vi "add channel test.vi"() -> (0 "no error":errorcluster, 1 "names":string[](array[string]), 2 "channels":refnum<class "TBM channel.lvclass">[](array[class]), 3 "sample module configuration out":refnum<class "sample module configuration.lvclass">)   [LabVIEW 2013, in "sample module tests.lvlib"]
uses:
  sample module tests.lvlib
  channel/TBM channel.lvclass
  module/configuration/sample module configuration.lvclass
  channel/channel classification.ctl
  root configuration/TBM configuration.lvclass
panel:
  out "channels match":bool
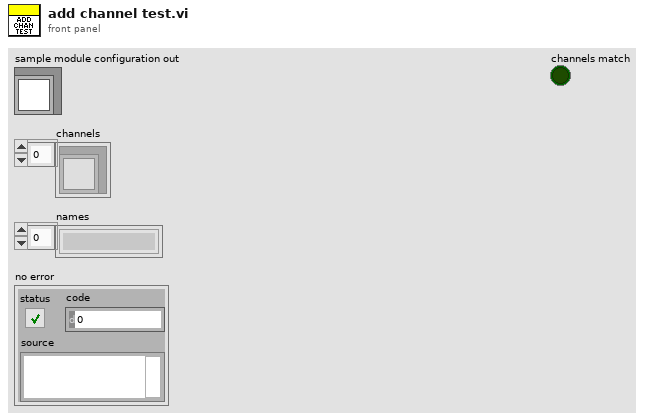
[diagram p1: front panel]
types:
  T1 = typedef "TBM channel.lvclass/channel classification.ctl" = enum16{"input data", "output data", "processing parameter", "processing result"}
  T2 = typedef "tag bus.lvlib/tag descriptor.lvclass/Data Type.ctl" = enum16{"Double", "Single", "I64", "I32", "I16", "I8", "U64", "U32", "U16", "U8", "Boolean", "String", "Array of Double", "Array of Single", "Array of I64", "Array of I32", "Array of I16", "Array of I8", "Array of U64", "Array of U32", "Array of U16", "Array of U8", "Array of Boolean", "Array of String"}
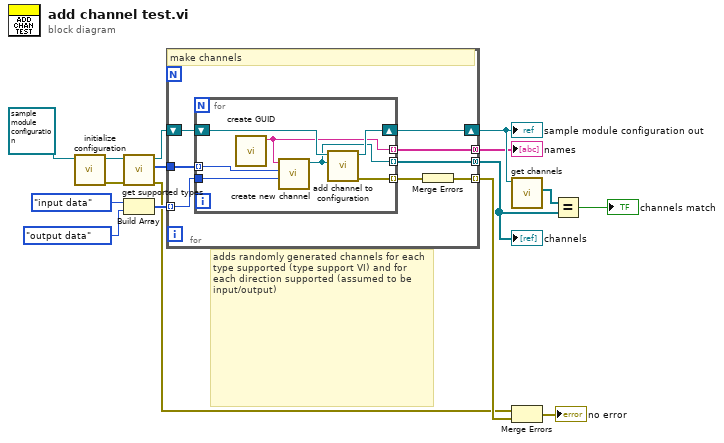
[diagram p0: block diagram]
diagram:
  # "adds randomly generated channels for each type supported (type support VI) and for each direction supported (assumed to be input/output)"
  n1 = call-dynamic "initialize configuration.vi"("configuration in"=refnum<class "sample module configuration.lvclass"> refnum ("sample module configuration")) -> ("error out"=w6:errorcluster, "configuration out"=w7:refnum<class "sample module configuration.lvclass">)  [unwired: 8 in, 1 out]
  n2 = call-dynamic "get supported types.vi"("error in"=w6, "sample module configuration in"=w7) -> ("error out"=w1:errorcluster, "supported types"=w4:T2[], "sample module configuration out"=w3:refnum<class "sample module configuration.lvclass">)  [unwired: 7 in]
  n3 = Build Array(channel_classification."input data" ("channel classification"), channel_classification."output data" ("channel classification")) -> (w14:T1[])
  n4 = for {
    tunnel: w14 -> [w24] mode=indexing
    tunnel: w4 -> [w23]
    tunnel: [w22] -> w11 mode=concatenating
    shift-right: [w20] -> w10
    shift-left: w3 -> [w21]
    tunnel: [w18] -> w9 mode=indexing
    tunnel: [w17] -> w2 mode=concatenating
    # "make channels"
    n5 = for {
      tunnel: w24 -> [w31]
      tunnel: w23 -> [w30] mode=indexing
      tunnel: [w27] -> w22 mode=indexing
      shift-right: [w28] -> w20
      shift-left: w21 -> [w29]
      tunnel: [w26] -> w19 mode=indexing
      tunnel: [w25] -> w17 mode=indexing
      n6 = call "create GUID.vi"() -> ("uuid"=w25:string)  [unwired: 11 in]
      n7 = call "create new channel.vi"("channel classification"=w31, "data type"=w30, "channel name"=w25) -> ("channel"=w27:refnum<class "TBM channel.lvclass">)  [unwired: 8 in]
      n8 = call "add channel to configuration.vi"("channel"=w27, "sample module configuration in"=w29) -> ("error out"=w26:errorcluster, "sample module configuration out"=w28:refnum<class "sample module configuration.lvclass">)  [unwired: 8 in]
    }
    n9 = Merge Errors(w19) -> (w18:errorcluster)
  }
  "channels" <- w11
  "sample module configuration out" <- w10
  "names" <- w2
  n10 = call-dynamic "get channels.vi"("module configuration in"=w10) -> ("channels"=w13:refnum<class "TBM channel.lvclass">[])  [unwired: 9 in, 1 out]
  n11 = Merge Errors(w1, w9) -> (→"no error":errorcluster)
  n12 = Equal?(x=w13, y=w11) -> (x = y?=→"channels match":bool)
